vi "test_Determine Trigger.vi"(8 "error in (no error)":errorcluster, 11 "TestCase in":refnum<class "Determine Trigger Unit Tests.lvclass">) -> (0 "error out":errorcluster, 3 "TestCase out":refnum<class "Determine Trigger Unit Tests.lvclass">)   [LabVIEW 2019, in "Determine Trigger Unit Tests.lvclass"]
uses:
  Determine Trigger Unit Tests.lvclass
  Addon/Addon Shared/Types/Command Channel Indeces.ctl
  Addon/Addon Shared/Types/Command Channel Index.ctl
  Addon/Addon Shared/Types/Message Parameters.ctl
  Addon/Addon Shared/Types/Message Generation Type.ctl
  <vilib>/addons/_JKI Toolkits/VI Tester/TestCase.llb/TestCase.lvclass
  Addon/Addon Engine/Instrument Addon Engine.lvlib
  Addon/Addon Shared/Instrument Addon Shared.lvlib
  C:/Program Files (x86)/National Instruments/LabVIEW 2019/vi.lib/addons/_JKI Toolkits/VI Tester/TestCase.llb/TestCase.lvclass
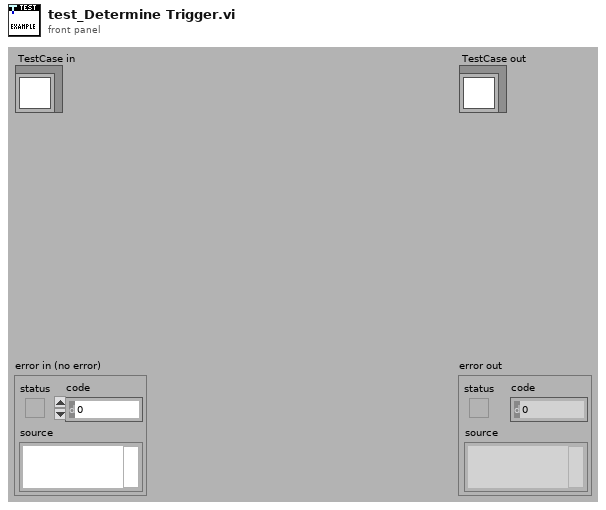
[diagram p1: front panel]
types:
  T1 = typedef "Instrument Addon Shared.lvlib/Message Generation Type.ctl" = enum16{"Trigger Only", "Periodic & Trigger", "Value Change & Trigger"}
  T2 = typedef "Instrument Addon Shared.lvlib/Command Channel Indeces.ctl" = cluster{"Channels":T3[]}
  T3 = typedef "Instrument Addon Shared.lvlib/Command Channel Index.ctl" = cluster{"Data Index":i32, "Data Length":i32}
  T4 = typedef "Instrument Addon Shared.lvlib/Message Parameters.ctl" = cluster{"Generation Type":T1, "Period":dbl, "Include Protection":bool, "Type":string}
  T5 = cluster{"Trigger":bool, "Command Indeces":T2, "Detect?":bool[], "Enabled":i32, "Time Since Last Generation":u32, "Message Parameters":T4}
  T6 = cluster{"Trigger":bool, "Command Indeces":T2, "Detect?":bool[], "Enabled":i32, "Time Since Last Generation":u32, "Message Parameters":T4}[]
  T7 = cluster{"Trigger":bool, "Time Since Last Generation":u32}
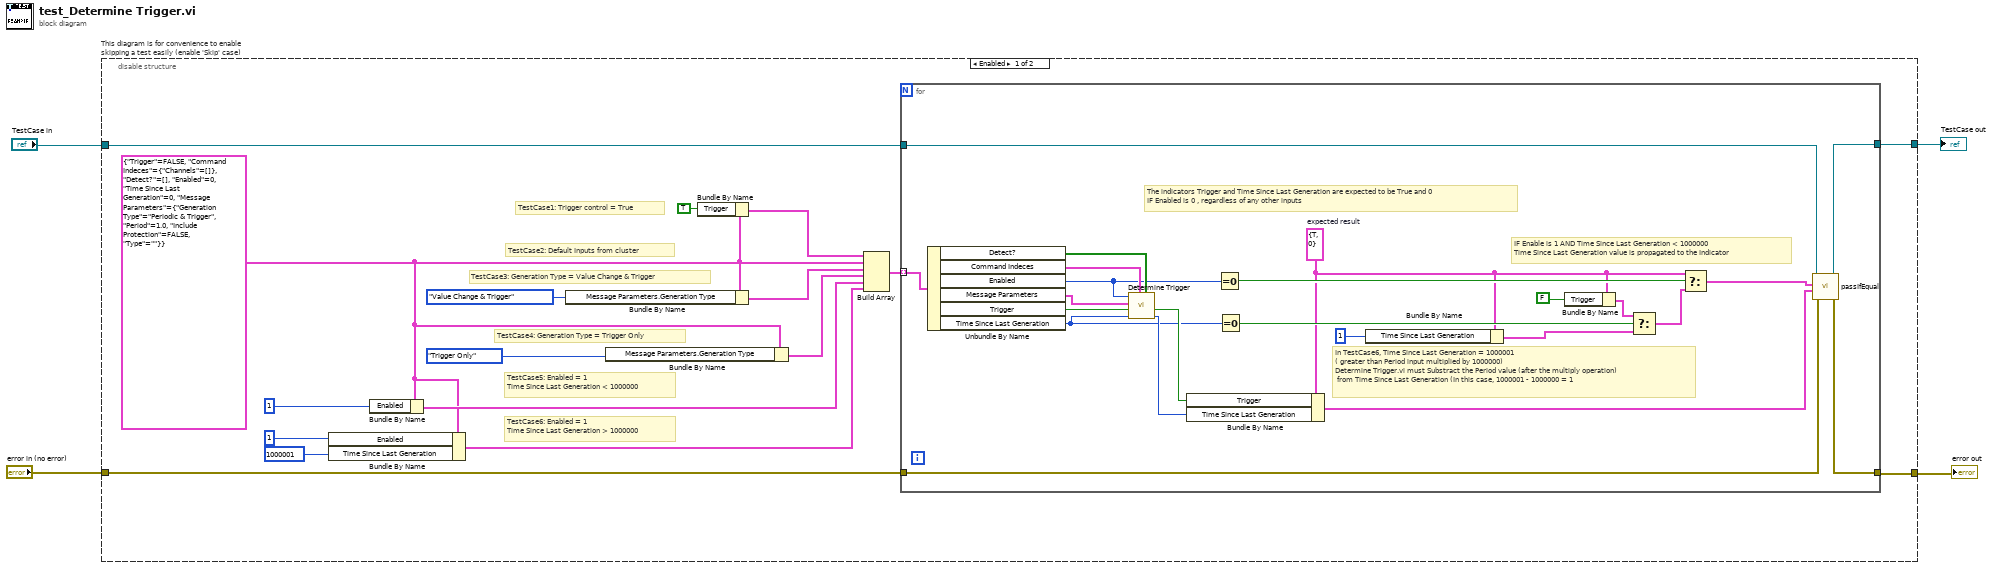
[diagram p0: block diagram]
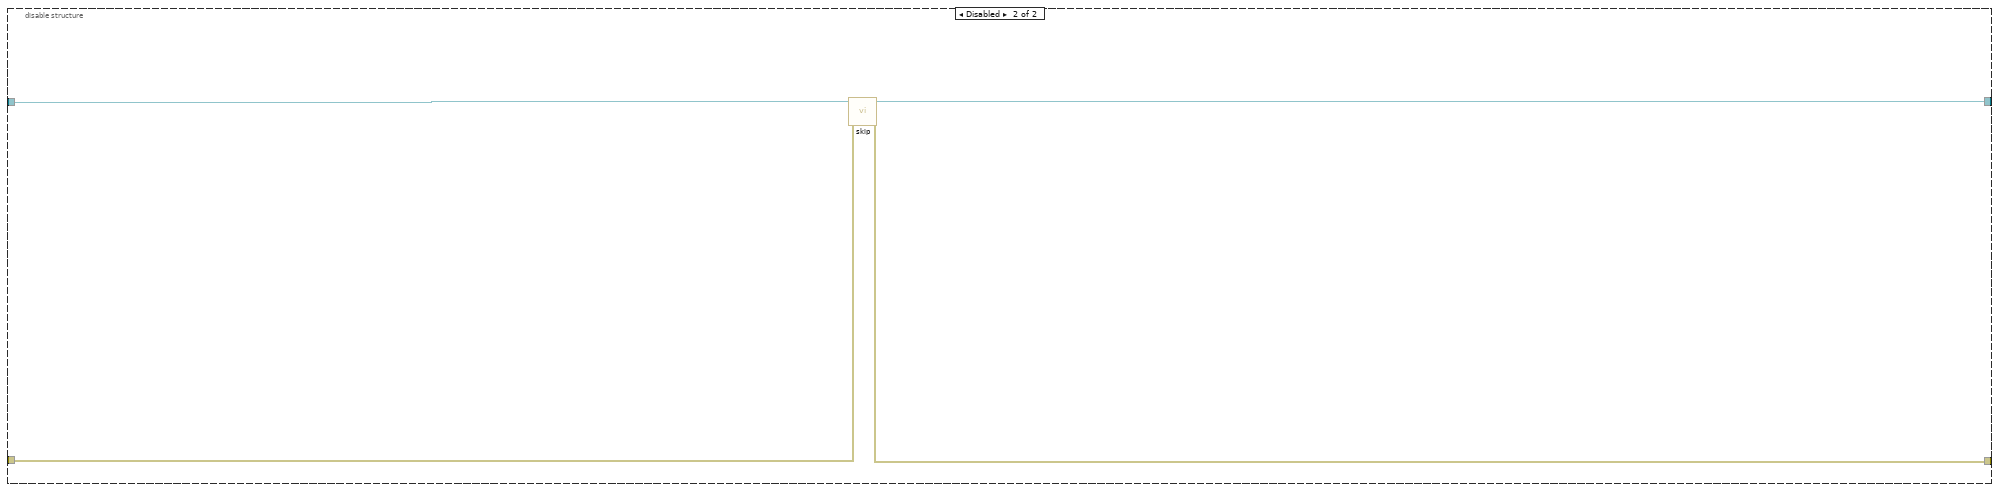
[diagram p2: hidden frame]
diagram:
  n1 = disable-structure "This diagram is for convenience to enable skipping a test easily (enable 'Skip' case)" shown="Enabled" {
    disable-tunnel: "TestCase in" -> [w21 w48]
    disable-tunnel: [w20 w46] -> w1
    disable-tunnel: [w19 w47] -> w3
    disable-tunnel: "error in (no error)" -> [w18 w45]
    frame Enabled {
      w5 = T5 {"Trigger"=FALSE, "Command Indeces"={"Channels"=[]}, "Detect?"=[], "Enabled"=0, "Time Since Last Generation"=0, "Message Parameters"={"Generation Type"=enum."Periodic & Trigger", "Period"=1.0, "Include Protection"=FALSE, "Type"=""}} ("Cluster")
      # "TestCase6: Enabled = 1\nTime Since Last Generation > 1000000"
      # "TestCase5: Enabled = 1\nTime Since Last Generation < 1000000"
      # "TestCase3: Generation Type = Value Change & Trigger"
      # "TestCase4: Generation Type = Trigger Only"
      # "TestCase2: Default Inputs from cluster"
      # "TestCase1: Trigger control = True"
      n2 = Bundle By Name(cluster=w5, "Enabled"=1, "Time Since Last Generation"=u32 1000001) -> (w6:T5)
      n3 = Bundle By Name(cluster=w5, "Enabled"=1) -> (w8:T5)
      n4 = Bundle By Name(cluster=w5, "Message Parameters.Generation Type"=Message_Generation_Type."Value Change & Trigger") -> (w11:T5)
      n5 = Bundle By Name(cluster=w5, "Message Parameters.Generation Type"=Message_Generation_Type."Trigger Only") -> (w10:T5)
      n6 = Bundle By Name(cluster=w5, "Trigger"=TRUE) -> (w16:T5)
      n7 = Build Array(w16, w5, w11, w10, w8, w6) -> (w15:T6)
      n8 = for {
        tunnel: w21 -> [w42]
        tunnel: [w40] -> w20
        tunnel: w18 -> [w43]
        tunnel: [w41] -> w19
        tunnel: w15 -> [w44] mode=indexing
        w24 = T7 {"Trigger"=TRUE, "Time Since Last Generation"=0}  # expected result
        # "IF Enable is 1 AND Time Since Last Generation < 1000000\nTime Since Last Generation value is propagated to the Indicator"
        # "In TestCase6, Time Since Last Generation = 1000001 \n( greater than Period input multiplied by 1000000)\nDetermine Trigger.vi must Substract the Period value (after the multiply operation)\n from Time Since Last Generation (In this case, 1000001 - 1000000 = 1"
        # "The indicators Trigger and Time Since Last Generation are expected to be True and 0 \nIF Enabled is 0 , regardless of any other inputs"
        n9 = Unbundle By Name(w44) -> ("Detect?"=w39:bool[], "Command Indeces"=w38:T2, "Enabled"=w32:i32, "Message Parameters"=w36:T4, "Trigger"=w37:bool, "Time Since Last Generation"=w28:u32)
        n10 = call "Determine Trigger.vi"("Detect?"=w39, "Command Indeces"=w38, "Time Since Last Generation"=w28, "Trigger"=w37, "Message Parameters"=w36, "Enabled"=w32) -> ("Time Since Last Generation"=w34:u32, "Trigger"=w35:bool)  [unwired: 4 in]
        n11 = Bundle By Name(cluster=w24, "Trigger"=w35, "Time Since Last Generation"=w34) -> (w33:T7)
        n12 = Equal To 0?(x=w32) -> (x = 0?=w31:bool)
        n13 = Equal To 0?(x=w28) -> (x = 0?=w27:bool)
        n14 = Bundle By Name(cluster=w24, "Time Since Last Generation"=u32 1) -> (w22:T7)
        n15 = Bundle By Name(cluster=w24, "Trigger"=FALSE) -> (w26:T7)
        n16 = Select(t=w26, s=w27, f=w22) -> (s? t:f=w25:T7)
        n17 = Select(t=w24, s=w31, f=w25) -> (s? t:f=w30:T7)
        n18 = call-dynamic "passIfEqual.vi"("error in (no error)"=w43, "y"=w33, "x"=w30, "TestCase in"=w42) -> ("error out"=w41:errorcluster, "TestCase out"=w40:refnum<class "Determine Trigger Unit Tests.lvclass">)  [unwired: 6 in]
      }
    }
    frame Disabled {
      # "skip test result while test is under development"
      n19 = call <vilib>:"skip.vi"("error in (no error)"=w45, "TestCase in"=w48) -> ("error out"=w47:errorcluster, "TestCase out"=w46:refnum<class "Determine Trigger Unit Tests.lvclass">)  [unwired: 8 in]
    }
  }
  "error out" <- w3
  "TestCase out" <- w1
